vi "Test 100000 Log Writes.vi"(11 "Test Case In":refnum<class "Stability.lvclass">) -> (0 "error out":errorcluster, 3 "Test Case Out":refnum<class "Stability.lvclass">)   [LabVIEW 2020, in "Stability.lvclass"]
uses:
  Stability.lvclass
  C:/Program Files (x86)/National Instruments/LabVIEW 2020/vi.lib/Astemes/LUnit/Test Case.lvclass
  Source/Type Defs/Debug Level.ctl
  <vilib>/Astemes/LUnit/Test Case.lvclass/Test Case.ctl
  a62785b1-2bf5-41ef-9482-6dbe5c31c84b.vi
  99935872-1fb4-4a94-a6a0-e8855ff45bf7.vi
  <vilib>/Astemes/LUnit/Core/LUnit Test Case/Private/Append Pass Result.vi
  <vilib>/Astemes/LUnit/Core/LUnit Test Case/Private/Append Fail Result.vi
  a62785b1-2bf5-41ef-9482-6dbe5c31c84b.vi/9c5d11cd-9439-4240-a1ee-d9baace9c924.vi
  99935872-1fb4-4a94-a6a0-e8855ff45bf7.vi/9c5d11cd-9439-4240-a1ee-d9baace9c924.vi
  <vilib>/Astemes/LUnit/Core/LUnit Test Case/Private/Run In UI.vi
  <vilib>/Utility/error.llb/Clear Errors.vi
  Source/Sinks/File Sink/File Sink.lvclass
  C:/Users/hughe_cx/Documents/05_repos/LVLog/Source/Sinks/Sink/Sink.lvclass
  Stability.lvclass/Stability.ctl
  Source/LV Log.lvlib
  Source/Logger/Logger.lvclass
  <vilib>/Astemes/LUnit/Test Case.lvclass
  C:/Users/hughe_cx/Documents/05_repos/LVLog/Source/Sinks/File Sink/File Sink.lvclass
  C:/Program Files (x86)/National Instruments/LabVIEW 2020/vi.lib/Astemes/LUnit/LUnit Runnable.lvclass
  C:/Users/hughe_cx/Documents/05_repos/LVLog/Testing/Stability/Stability.lvclass
panel:
  out "Iteration (of 100000)":i32
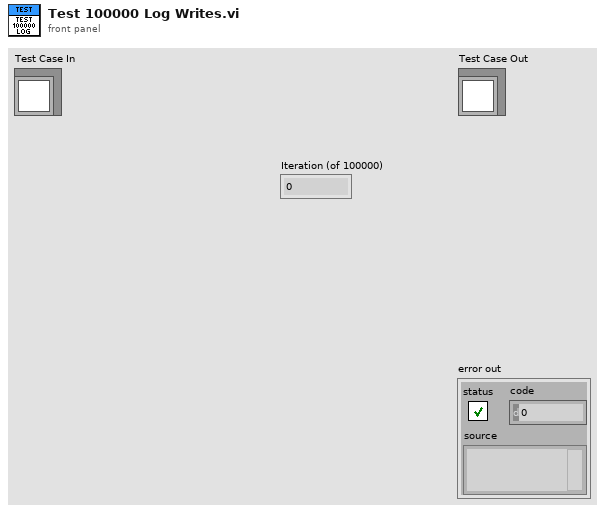
[diagram p1: front panel]
types:
  T1 = typedef "LV Log.lvlib/Debug Level.ctl" = enum16{"DEFAULT", "DEBUG", "INFO", "WARN", "ERROR", "FATAL"}
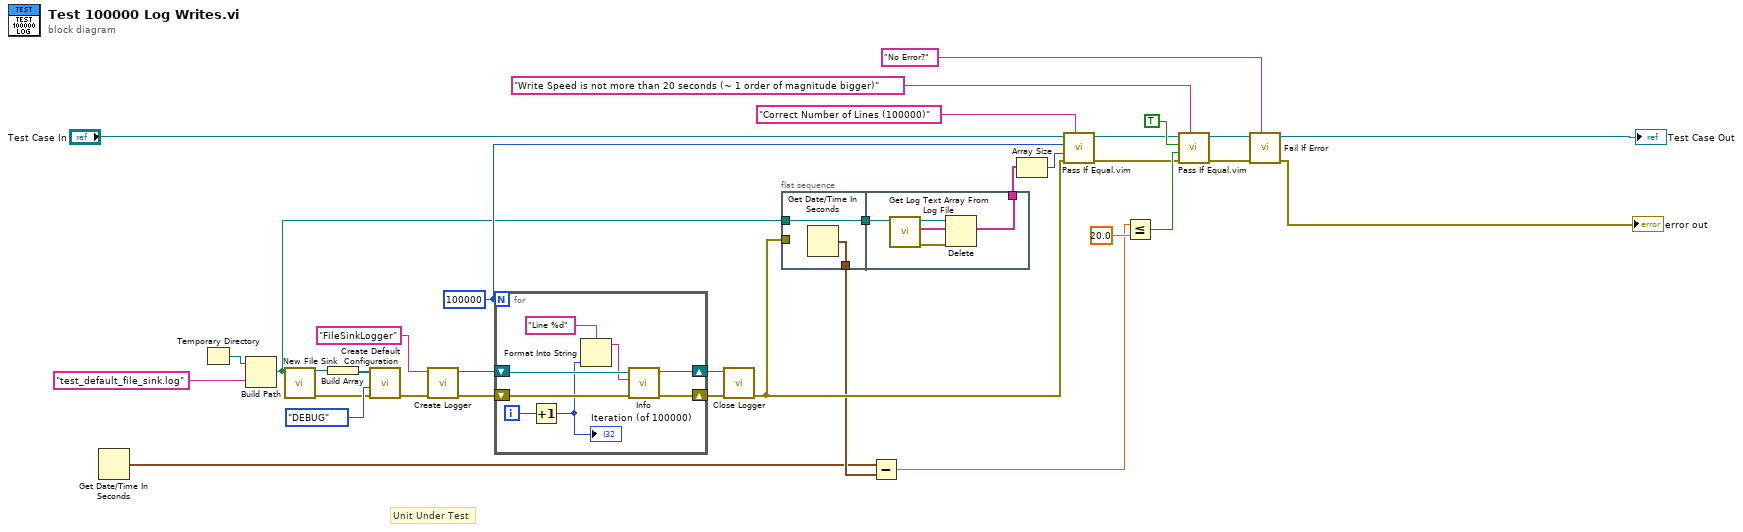
[diagram p0: block diagram]
diagram:
  w19 = 100000
  # "Unit Under Test"
  n1 = Get Date/Time In Seconds() -> (seconds since 1Jan1904=w24:timestamp)
  n2 = Temporary Directory() -> (w9:path)
  n3 = Build Path(base path=w9, name or relative path="test_default_file_sink.log" ("format string")) -> (appended path=w14:path)
  n4 = call "New File Sink.vi"("File Path"=w14) -> ("error out"=w6:errorcluster, "File Sink out"=w8:refnum<class "File Sink.lvclass">)  [unwired: 9 in]
  n5 = Build Array(w8) -> (w7:refnum<class "File Sink.lvclass">[])
  n6 = call "Create Default Configuration.vi"("Sinks"=w7, "Debug Level in"=Debug_Level."DEBUG", "error in (no error)"=w6) -> ("error out"=w5:errorcluster)  [unwired: 7 in]
  n7 = call "Create Logger.vi"("error in (no error)"=w5, "Name"="FileSinkLogger") -> ("error out"=w11:errorcluster, "Logger out"=w12:refnum<class "Logger.lvclass">)  [unwired: 8 in]
  n8 = for {
    N: w19 -> [_]
    shift-right: [w39] -> w31
    shift-left: w12 -> [w41]
    shift-right: [w40] -> w32
    shift-left: w11 -> [w42]
    i -> [w36]
    n9 = Increment(x=w36) -> (x+1=w35:i32)
    "Iteration (of 100000)" <- w35
    n10 = Format Into String(format string="Line %d" ("Log Text"), w35) -> (resulting string=w37:string)  [unwired: 2 in, 1 out]
    n11 = call "Info.vi"("error in (no error)"=w42, "Log Text"=w37, "Logger in"=w41) -> ("error out"=w40:errorcluster, "Logger out"=w39:refnum<class "Logger.lvclass">)  [unwired: 6 in, 1 out]
  }
  n12 = call "Close Logger.vi"("error in (no error)"=w32, "Logger in"=w31) -> ("error out"=w33:errorcluster)  [unwired: 9 in]
  n13 = flat-sequence {
    tunnel: w33 -> [_]
    tunnel: w14 -> [w44]
    tunnel: [w44] -> w34
    tunnel: [w43] -> w25
    tunnel: [w48] -> w15
    tunnel: w34 -> [w47]
    frame #0 {
      n14 = Get Date/Time In Seconds() -> (seconds since 1Jan1904=w43:timestamp)
    }
    frame #1 {
      n15 = call "Get Log Text Array From Log File.vi"("Log File Path in"=w47) -> ("error out"=w45:errorcluster, "Log Text Array"=w48:string[], "Log File Path out"=w46:path)  [unwired: 8 in]
      n16 = Delete(path (use dialog)=w46, error in=w45) -> ()  [unwired: 3 in, 3 out]
    }
  }
  n17 = Subtract(x=w24, y=w25) -> (x-y=w27:dbl)
  n18 = Array Size(array=w15) -> (size(s)=w16:i32)
  n19 = call "Pass If Equal.vim"("Description"="Correct Number of Lines (100000)", "error in (no error)"=w33, "Actual"=w16, "Expected"=w19, "LUnit Test Case In"="Test Case In") -> ("error out"=w22:errorcluster, "LUnit Test Case Out"=w20:refnum<class "Stability.lvclass">)  [unwired: 5 in]
  n20 = Less Or Equal?(x=w27, y=20.0) -> (x <= y?=w29:bool)
  n21 = call "Pass If Equal.vim"("Description"="Write Speed is not more than 20 seconds (~ 1 order of magnitude bigger)", "error in (no error)"=w22, "Actual"=w29, "Expected"=TRUE, "LUnit Test Case In"=w20) -> ("error out"=w23:errorcluster, "LUnit Test Case Out"=w21:refnum<class "Stability.lvclass">)  [unwired: 5 in]
  n22 = call <vilib>:"Fail If Error.vi"("Description"="No Error?", "error in (no error)"=w23, "LUnit Test Case In"=w21) -> ("error out"=→"error out":errorcluster, "LUnit Test Case Out"=→"Test Case Out":refnum<class "Stability.lvclass">)  [unwired: 7 in]
